vi "String to U16.vi"(5 "Array of Strings":string[](array[string])) -> (2 "Array of U16":u16[](array[numeric]) format="%x")   [LabVIEW 2021, in "Update Enum.lvlib"]
doc: "This Vi convert a array of string in a array of V16 \n rules : each string is preceed by the number of characters follow-up by the ascii value of all of it. And all the blocks (Number+ascii code) are grouped and truncated in V16 array data.\nNote : if there is not enough characters a last 00 is add. \n\nThis convertion is usefull for typeDescriptor Data\n\nEric Bobillier INRA15/01/2007 France (eric.bobillier@rennes.inra.fr)"
uses:
  Update Enum.lvlib
panel:
  # "This Vi convert a array of string in a array of U16 \n rules : each string is preceed by the number of characters follow-up by the ascii value of all of it. \nAnd all the blocks (Number+ascii code) are grouped and truncated in U16 array data.\nNote : if there is not enough characters a last 00 is add. \n\nThis convertion is usefull for typeDescriptor Data\n\nEric Bobillier INRA15/01/2007  France   (eric.bobillier@rennes.inra.fr)"
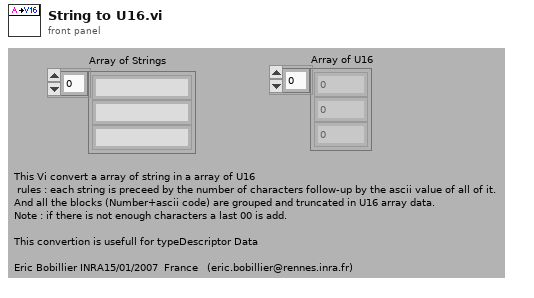
[diagram p1: front panel]
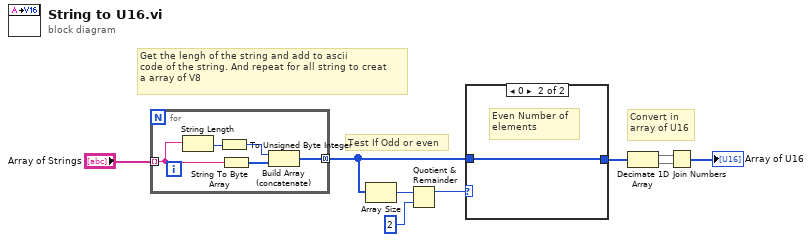
[diagram p0: block diagram]
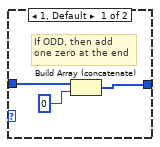
[diagram p2: hidden frame]
diagram:
  # "Convert in \narray of U16"
  # "Test If Odd or even"
  # "Get the lengh of the string and add to ascii \ncode of the string. And repeat for all string to creat\na array of V8"
  n1 = for {
    tunnel: "Array of Strings" -> [w13] mode=indexing
    tunnel: [w10] -> w4 mode=concatenating
    n2 = String Length(string=w13) -> (length=w14:i32)
    n3 = To Unsigned Byte Integer(number=w14) -> (unsigned 8bit integer=w12:u8)
    n4 = String To Byte Array(string=w13) -> (unsigned byte array=w11:u8[])
    n5 = Build Array (concatenate)(w12, w11) -> (w10:u8[])
  }
  n6 = Array Size(array=w4) -> (size(s)=w5:i32)
  n7 = Quotient & Remainder(x=w5, y=2) -> (x-y*floor(x/y)=w3:i32)  [unwired: 1 out]
  n8 = case shown="0" w3 {
    tunnel: [w15 w18] -> w9
    tunnel: w4 -> [w16 w18]
    frame 1, Default {
      # "If ODD, then add \none zero at the end"
      n9 = Build Array (concatenate)(w16, u8 0) -> (w15:u8[])
    }
    frame 0 {
      # "Even Number of\nelements"
    }
  }
  n10 = Decimate 1D Array(w9) -> (w7:u8[], w8:u8[])
  n11 = Join Numbers(hi=w7, lo=w8) -> ((hi.lo)=→"Array of U16":u16[])
